vi "1RowDataToArrayofVData.vi"(6 "Header":string[](array[string]), 7 "HeaderPrefix":string, 8 "error in (no error)":errorcluster, 10 "Data in":string[](array[string]), 11 "Variant":variant) -> (0 "error out":errorcluster, 3 "Varaint Out":variant)   [LabVIEW 2014, in "TableLogger_Actor.lvlib" / "TableLogger_Actor.lvclass"]
uses:
  TableLogger_Actor.lvclass
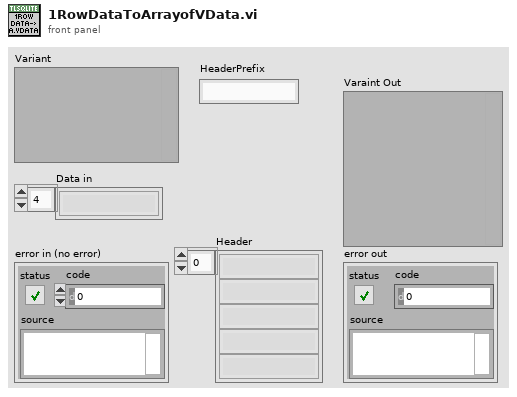
[diagram p1: front panel]
types:
  T1 = typedef "Type Descriptor Enumeration__ogtk.ctl" = enum8{"<Null>", "I8", "I16", "I32", "I64", "U8", "U16", "U32", "U64", "SGL", "DBL", "EXT", "CSG", "CDB", "CXT", "0x0F", "0x10", "0x11", "0x12", "0x13", "0x14", "Enum U8", "Enum U16", "Enum U32", "Enum U64", "SGL PQ", "DBL PQ", "EXT PQ", "CSG PQ", "CDB PQ", "CXT PQ", "0x1F", "0x20", "Boolean", "0x22", "0x23", "0x24", "0x25", "0x26", "0x27", "0x28", "0x29", "0x2A", "0x2B", "0x2C", "0x2D", "0x2E", "0x2F", "String", "0x31", "Path", "Pict", "0x34", "0x35", "0x36", "DAQ", "0x38", "0x39", "0x3A", "0x3B", "0x3C", "0x3D", "0x3E", "0x3F", "Array", "0x41", "0x42", "0x43", "0x44", "0x45", "0x46", "0x47", "0x48", "0x49", "0x4A", "0x4B", "0x4C", "0x4D", "0x4E", "0x4F", "Cluster", "0x51", "0x52", "Variant", "Waveform", "0x55", "0x56", "0x57", "0x58", "0x59", "0x5A", "0x5B", "0x5C", "0x5D", "0x5E", "0x5F", "0x60", "0x61", "0x62", "0x63", "0x64", "0x65", "0x66", "0x67", "0x68", "0x69", "0x6A", "0x6B", "0x6C", "0x6D", "0x6E", "0x6F", "Refnum"}
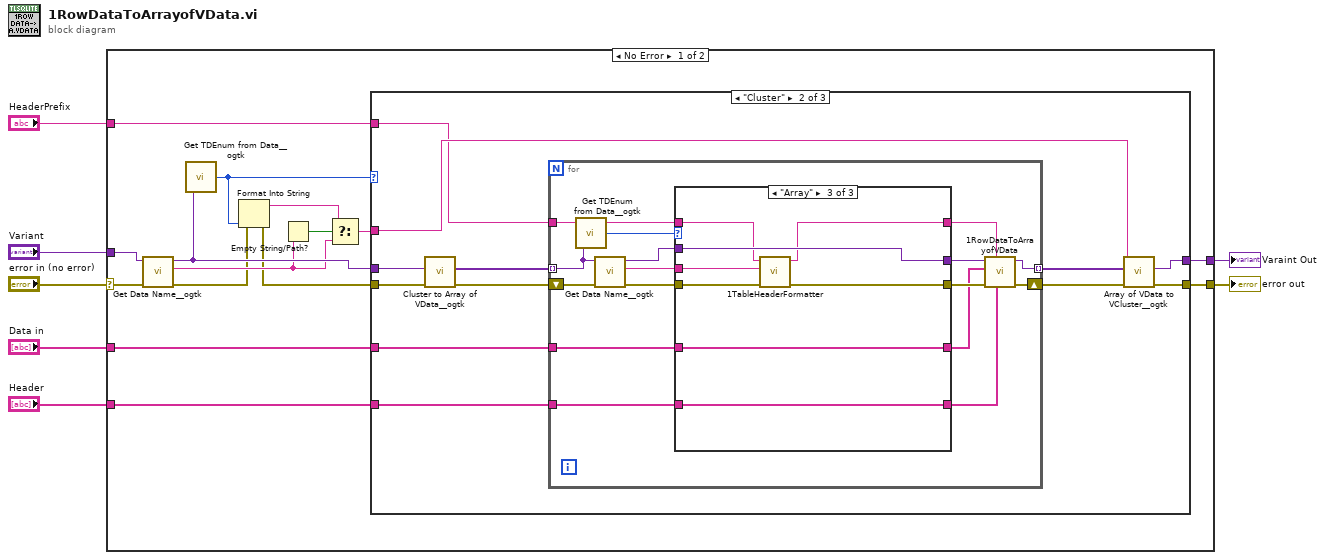
[diagram p0: block diagram]
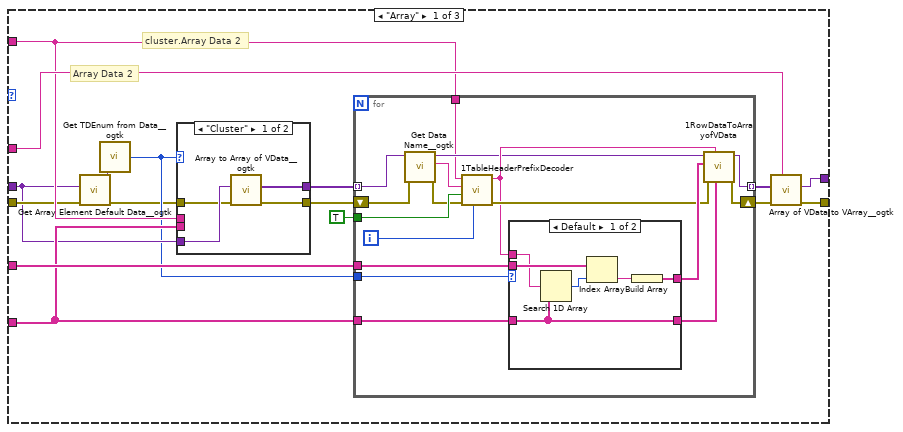
[diagram p2: hidden frame]
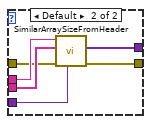
[diagram p3: hidden frame]
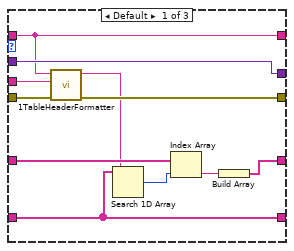
[diagram p5: hidden frame]
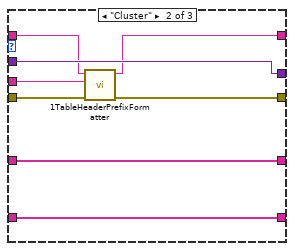
[diagram p6: hidden frame]
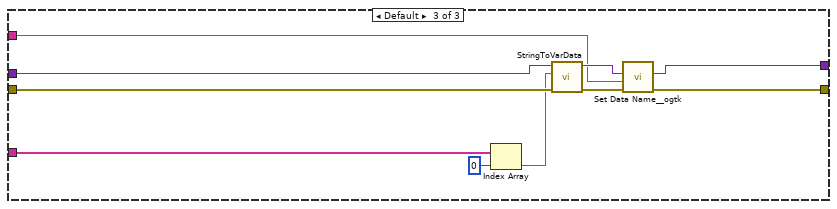
[diagram p7: hidden frame]
diagram:
  n1 = case shown="No Error" "error in (no error)" {
    selector: "error in (no error)" -> [w15 w139]
    tunnel: "Data in" -> [w20 _]
    tunnel: "Variant" -> [w16 _]
    tunnel: [w22 w139] -> w6
    tunnel: [w21 _] -> w5
    tunnel: "Header" -> [w19 _]
    tunnel: "HeaderPrefix" -> [w8 _]
    frame No Error {
      n2 = call <userlib>:"Get Data Name__ogtk.vi"("error in (no error)"=w15, "Data"=w16) -> ("error out"=w10:errorcluster, "Data Name"=w11:string, "Data dup"=w14:variant)  [unwired: 7 in]
      n3 = call <userlib>:"Get TDEnum from Data__ogtk.vi"("Data"=w14) -> ("Type Descriptor Enumeration"=w13:T1)  [unwired: 4 in]
      n4 = Format Into String(error in=w10, w13) -> (resulting string=w18:string, error out=w9:errorcluster)  [unwired: 2 in]
      n5 = Empty String/Path?(string/path=w11) -> (empty?=w17:bool)
      n6 = Select(t=w18, s=w17, f=w11) -> (s? t:f=w12:string)
      n7 = case shown="\"Cluster\"" w13 {
        tunnel: w14 -> [w26 w82 w138]
        tunnel: [w38 w84 w136] -> w21
        tunnel: w9 -> [w30 w83 w133]
        tunnel: [w31 w85 w134] -> w22
        tunnel: w20 -> [w36 w79 w132]
        tunnel: w19 -> [w33 w78 _]
        tunnel: w12 -> [w35 w75 w129]
        tunnel: w8 -> [w32 w74 _]
        frame "Array" {
          # "Array Data 2"
          # "cluster.Array Data 2"
          n8 = call <userlib>:"Get Array Element Default Data__ogtk.vi"("error in (no error)"=w30, "Array"=w26) -> ("error out"=w24:errorcluster, "Array Element Default Data"=w23:variant)  [unwired: 8 in]
          n9 = call <userlib>:"Get TDEnum from Data__ogtk.vi"("Data"=w23) -> ("Type Descriptor Enumeration"=w25:T1)  [unwired: 4 in]
          n10 = case shown="\"Cluster\"" w25 {
            tunnel: w33 -> [_ w48]
            tunnel: w32 -> [_ w47]
            tunnel: w24 -> [w41 w45]
            tunnel: [w40 w46] -> w28
            tunnel: [w39 w44] -> w27
            tunnel: w26 -> [w42 w43]
            frame "Cluster" {
              n11 = call <userlib>:"Array to Array of VData__ogtk.vi"("error in (no error)"=w41, "MultiD Array"=w42) -> ("error out"=w39:errorcluster, "1D Array of Variants"=w40:variant[])  [unwired: 8 in]
            }
            frame Default {
              n12 = call "SimilarArraySizeFromHeader.vi"("Array Element Data"=w43, "error in (no error)"=w45, "Headers"=w48, "Prefix Name"=w47) -> ("error out"=w44:errorcluster, "1D Array of Variants Initialized"=w46:variant[])  [unwired: 6 in]
            }
          }
          n13 = for {
            shift-right: [w65] -> w37
            shift-left: w27 -> [w59]
            tunnel: w28 -> [w53] mode=indexing
            tunnel: [w52] -> w34 mode=indexing
            tunnel: w36 -> [w64]
            tunnel: w33 -> [w50]
            tunnel: TRUE -> [w62]
            tunnel: w32 -> [w55]
            tunnel: w25 -> [w51]
            i -> [w54]
            n14 = call <userlib>:"Get Data Name__ogtk.vi"("error in (no error)"=w59, "Data"=w53) -> ("error out"=w58:errorcluster, "Data Name"=w56:string, "Data dup"=w57:variant)  [unwired: 7 in]
            n15 = call "1TableHeaderPrefixDecoder.vi"("ArrayIndex"=w54, "error in"=w58, "Array?"=w62, "Added HeaderPrefix"=w56, "Existing HeaderPrefix"=w55) -> ("error out"=w61:errorcluster, "HeaderPrefix"=w60:string)  [unwired: 5 in]
            n16 = case shown="Default" w51 {
              tunnel: w64 -> [w70 w73]
              tunnel: [w68 w73] -> w63
              tunnel: w60 -> [w67 _]
              tunnel: w50 -> [w66 w72]
              tunnel: [w66 w72] -> w49
              frame Default {
                n17 = Search 1D Array(1D array=w66, element=w67) -> (index of element=w71:i32)  [unwired: 1 in]
                n18 = Index Array(array=w70, index=w71) -> (element=w69:string)
                n19 = Build Array(w69) -> (w68:string[])
              }
              frame "Cluster" {
              }
            }
            n20 = call "1RowDataToArrayofVData.vi"("Header"=w49, "HeaderPrefix"=w60, "error in (no error)"=w61, "Data in"=w63, "Variant"=w57) -> ("error out"=w65:errorcluster, "Varaint Out"=w52:variant)  [unwired: 5 in]
          }
          n21 = call <userlib>:"Array of VData to VArray__ogtk.vi"("Array Name"=w35, "error in (no error)"=w37, "1D Array of VData"=w34) -> ("error out"=w31:errorcluster, "VArray"=w38:variant)  [unwired: 7 in]
        }
        frame "Cluster" {
          n22 = call <userlib>:"Cluster to Array of VData__ogtk.vi"("error in (no error)"=w83, "Cluster"=w82) -> ("error out"=w80:errorcluster, "Array of VData"=w81:variant[])  [unwired: 8 in]
          n23 = for {
            shift-right: [w94] -> w76
            shift-left: w80 -> [w100]
            tunnel: w81 -> [w98] mode=indexing
            tunnel: [w92] -> w77 mode=indexing
            tunnel: w79 -> [w91]
            tunnel: w78 -> [w90]
            tunnel: w74 -> [w87]
            n24 = call <userlib>:"Get TDEnum from Data__ogtk.vi"("Data"=w98) -> ("Type Descriptor Enumeration"=w101:T1)  [unwired: 4 in]
            n25 = call <userlib>:"Get Data Name__ogtk.vi"("error in (no error)"=w100, "Data"=w98) -> ("error out"=w99:errorcluster, "Data Name"=w96:string, "Data dup"=w97:variant)  [unwired: 7 in]
            n26 = case shown="\"Array\"" w101 {
              tunnel: [w104 w116 w124] -> w95
              tunnel: [w112 w120 w128] -> w93
              tunnel: w99 -> [w105 w117 w125]
              tunnel: w97 -> [w112 w120 w128]
              tunnel: w96 -> [w106 w114 w123]
              tunnel: w91 -> [w109 w119 w127]
              tunnel: w90 -> [w107 w118 w126]
              tunnel: [w108 w119 w127] -> w89
              tunnel: [w107 w118 w126] -> w88
              tunnel: w87 -> [w102 w115 w122]
              tunnel: [w102 w113 w121] -> w86
              frame Default {
                n27 = call "1TableHeaderFormatter.vi"("error in (no error)"=w105, "Data Name"=w106, "HeaderPrefix"=w102) -> ("error out"=w104:errorcluster, "HeaderOut"=w103:string)  [unwired: 7 in]
                n28 = Search 1D Array(1D array=w107, element=w103) -> (index of element=w111:i32)  [unwired: 1 in]
                n29 = Index Array(array=w109, index=w111) -> (element=w110:string)
                n30 = Build Array(w110) -> (w108:string[])
              }
              frame "Cluster" {
                n31 = call "1TableHeaderPrefixFormatter.vi"("error in"=w117, "Added HeaderPrefix"=w114, "Existing HeaderPrefix"=w115) -> ("error out"=w116:errorcluster, "HeaderPrefix"=w113:string)  [unwired: 7 in]
              }
              frame "Array" {
                n32 = call "1TableHeaderFormatter.vi"("error in (no error)"=w125, "Data Name"=w123, "HeaderPrefix"=w122) -> ("error out"=w124:errorcluster, "HeaderOut"=w121:string)  [unwired: 7 in]
              }
            }
            n33 = call "1RowDataToArrayofVData.vi"("Header"=w88, "HeaderPrefix"=w86, "error in (no error)"=w95, "Data in"=w89, "Variant"=w93) -> ("error out"=w94:errorcluster, "Varaint Out"=w92:variant)  [unwired: 5 in]
          }
          n34 = call <userlib>:"Array of VData to VCluster__ogtk.vi"("error in (no error)"=w76, "Cluster Name"=w75, "Array"=w77) -> ("error out"=w85:errorcluster, "VCluster"=w84:variant)  [unwired: 7 in]
        }
        frame Default {
          n35 = Index Array(array=w132, index=0) -> (element=w131:string)
          n36 = call "StringToVarData.vi"("error in (no error)"=w133, "String Value"=w131, "Variant ref"=w138) -> ("error out"=w135:errorcluster, "Varaint Out"=w137:variant)  [unwired: 7 in]
          n37 = call <userlib>:"Set Data Name__ogtk.vi"("error in (no error)"=w135, "Data Name"=w129, "Data"=w137) -> ("error out"=w134:errorcluster, "Renamed Data"=w136:variant)  [unwired: 7 in]
        }
      }
    }
    frame Error {
    }
  }
  "error out" <- w6
  "Varaint Out" <- w5
